vi "AOL Z Cal-Optimised Z sequence.vi"(6 "Negative first (F)":bool, 9 "Max positive value":dbl=1.0 format="%#_13g", 11 "Calibration points":i32=21 min=5 max=100) -> (1 "Decending order":dbl[](array[numeric]), 3 "Calibration's optimised norm Z sequence":dbl[](array[numeric]))   [LabVIEW 2017]
panel:
  out "size(s)":i32
  out "Increment":dbl format="%#_12f"
  # "Recommended numbers of calibration points are 11, 21, 41 etc such as the increment step is always a nice value rounded to two decimal points."
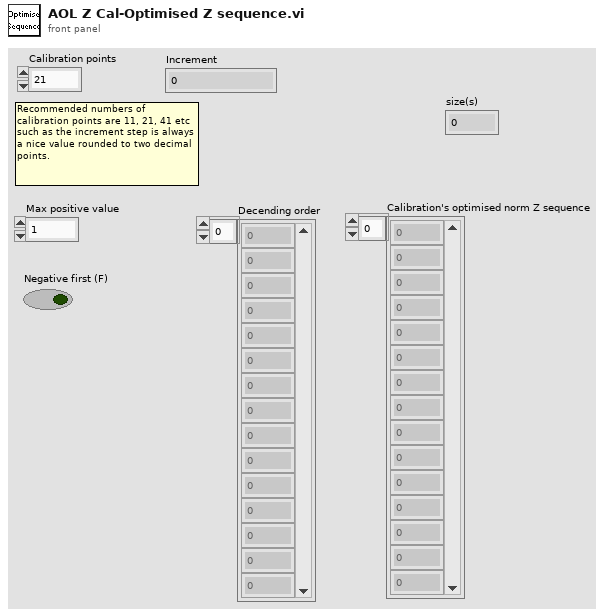
[diagram p1: front panel]
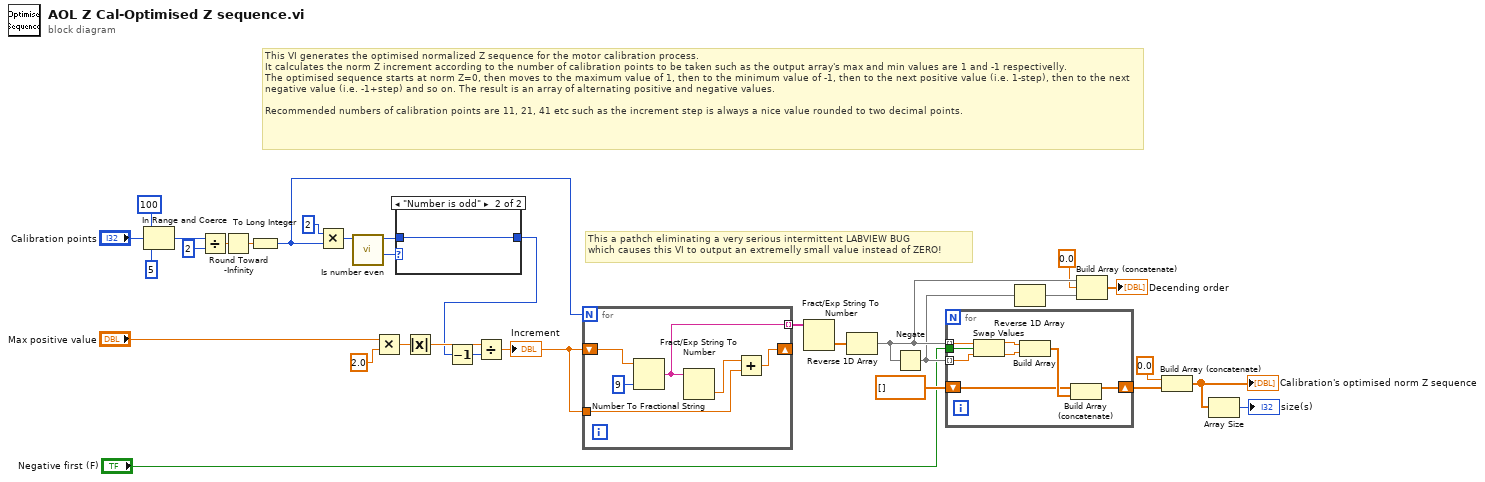
[diagram p0: block diagram]
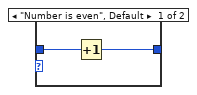
[diagram p2: hidden frame]
diagram:
  # "This VI generates the optimised normalized Z sequence for the motor calibration process.\nIt calculates the norm Z increment according to the number of calibration points to be taken such as the output array's max and min values are 1 and -1 respectivelly.\nThe optimised sequence starts at norm Z=0, then moves to the maximum value of 1, then to the minimum value of -1, then to the next positive value (i.e. 1-step), then to the next negative value (i.e. -1+step) and so on. The result is an array of alternating positive and negative values.\n\nRecommended numbers of calibration points are 11, 21, 41 etc such as the increment step is always a nice value rounded to two decimal points."
  # "This a pathch eliminating a very serious intermittent LABVIEW BUG\nwhich causes this VI to output an extremelly small value instead of ZERO!"
  n1 = In Range and Coerce(upper limit=100, x="Calibration points", lower limit=5) -> (coerced(x)=w12:i32)  [unwired: 1 out]
  n2 = Divide(x=w12, y=2) -> (x/y=w26:dbl)
  n3 = Round Toward -Infinity(1:w26) -> (0:w18:dbl)
  n4 = To Long Integer(number=w18) -> (32bit integer=w10:i32)
  n5 = Multiply(x=2, y=w10) -> (x*y=w9:i32)
  n6 = call "Is number even.vi"("Number"=w9) -> ("Even/Odd"=w32:enum16{"Number is even", "Number is odd"}, "Number (dup)"=w8:i32)  [unwired: 9 in]
  n7 = Multiply(x="Max positive value", y=2.0) -> (x*y=w24:dbl)
  n8 = case shown="\"Number is odd\"" w32 {
    tunnel: [w33 w35] -> w11
    tunnel: w8 -> [w34 w35]
    frame "Number is even", Default {
      n9 = Increment(x=w34) -> (x+1=w33:i32)
    }
    frame "Number is odd" {
    }
  }
  n10 = Absolute Value(x=w24) -> (abs(x)=w31:dbl)
  n11 = Decrement(x=w11) -> (x-1=w30:i32)
  n12 = Divide(x=w31, y=w30) -> (x/y=w28:dbl)
  "Increment" <- w28
  n13 = for {
    N: w10 -> [_]
    shift-right: [w40] -> _
    shift-left: w28 -> [w38]
    tunnel: w28 -> [w41]
    tunnel: [w36] -> w29 mode=indexing
    n14 = Number To Fractional String(number=w38, precision (6)=i16 9) -> (F-format string=w36:string)  [unwired: 2 in]
    n15 = Fract/Exp String To Number(string=w36) -> (number=w37:dbl)  [unwired: 3 in, 1 out]
    n16 = Add(x=w37, y=w41) -> (x+y=w40:dbl)
  }
  n17 = Fract/Exp String To Number(string=w29) -> (number=w22:dbl[])  [unwired: 3 in, 1 out]
  n18 = Reverse 1D Array(array=w22) -> (reversed array=w6:dbl[])
  n19 = Negate(x=w6) -> (-x=w5:dbl[])
  n20 = for {
    tunnel: w6 -> [w46] mode=indexing
    tunnel: w5 -> [w45] mode=indexing
    shift-right: [w48] -> w20
    shift-left: dbl[] [] -> [w47]
    tunnel: "Negative first (F)" -> [w42]
    n21 = Swap Values(12:w46, 13:w42, 14:w45) -> (1:w43:dbl, 3:w44:dbl)
    n22 = Build Array(w43, w44) -> (w49:dbl[])
    n23 = Build Array (concatenate)(w47, w49) -> (w48:dbl[])
  }
  n24 = Reverse 1D Array(array=w5) -> (reversed array=w3:dbl[])
  n25 = Build Array (concatenate)(w6, 0.0 ("x/y"), w3) -> (→"Decending order":dbl[])
  n26 = Build Array (concatenate)(0.0 ("x/y"), w20) -> (w17:dbl[])
  "Calibration's optimised norm Z sequence" <- w17
  n27 = Array Size(array=w17) -> (size(s)=→"size(s)":i32)
